vi "AlliGator Get Background Subtraction Parameters.vi"(6 "Get (F)/Set":bool, 8 "Error In":errorcluster, 11 "Background Subtraction Parameters in":T1={"Background Definition Range"={"Min Gate"=0.0, "Max Gate"=0.0}, "Baseline Subtraction Method"=enum."Mean", "Background Subtraction?"=FALSE, "Background File"=path "", "Background Constant"=0.0, "Background Scaling Factor"=1.0, "Background Pile-up Correction"=FALSE, "Background Pixel Well Capacity"=1} {"Background Pixel Well Capacity" min=1 step=1}) -> (0 "Error Out":errorcluster, 3 "Background Subtraction Parameters out":T1={"Background Definition Range"={"Min Gate"=0.0, "Max Gate"=0.0}, "Baseline Subtraction Method"=enum."Mean", "Background Subtraction?"=FALSE, "Background File"=path "", "Background Constant"=0.0, "Background Scaling Factor"=1.0, "Background Pile-up Correction"=FALSE, "Background Pixel Well Capacity"=1} {"Background Pixel Well Capacity" min=1 step=1})   [LabVIEW 2021, in "AlliGator Decay Preprocessing.lvlib"]
doc: "Obtains or stores information about <B>Background Subtraction Parameters</B> from Settings."
uses:
  AlliGator Decay Preprocessing.lvlib
  AlliGator Background Subtraction Parameters.ctl
  AlliGator Baseline Subtraction Method.ctl
  Settings/AlliGator Settings List.ctl
  Settings/AlliGator Settings.lvlib
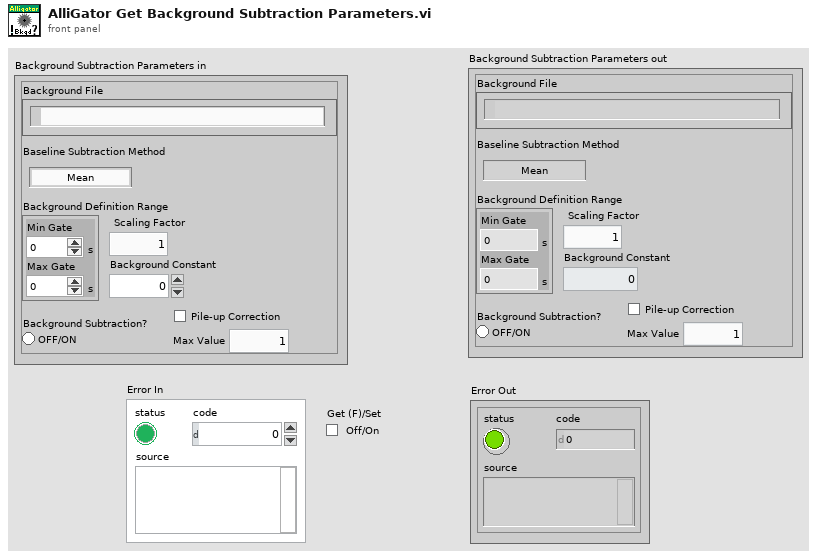
[diagram p1: front panel]
types:
  T1 = typedef "AlliGator Decay Preprocessing.lvlib/AlliGator Background Subtraction Parameters.ctl" = cluster{"Background Definition Range":cluster{"Min Gate":dbl[unit], "Max Gate":dbl[unit]}, "Baseline Subtraction Method":T2, "Background Subtraction?":bool, "Background File":path, "Background Constant":dbl, "Background Scaling Factor":dbl, "Background Pile-up Correction":bool, "Background Pixel Well Capacity":u32}
  T2 = typedef "AlliGator Decay Preprocessing.lvlib/AlliGator Baseline Subtraction Method.ctl" = enum16{"Mean", "Min", "Square Gated Single-Exponential", "File", "Constant"}
  T3 = typedef "AlliGator Settings.lvlib/AlliGator Settings List.ctl" = enum16{"GUI:Visible Settings Tab", "GUI:Last Run Version", "Source Image:Use Image Histogram for Contrast", "Source Image:Low Count Pixels Rejection Options", "Source Image:High Count Pixels Rejection Options", "Source Image:Use Image Brightness", "Source Image:Blend Overlay with Image Background", "Source Image:Use Fixed ROI Diameter", "Source Image:ROI Diameter", "Source Image:ROI Center Color", "Source Image:Peak Threshold", "Source Image:Intensity Threshold", "Source Image:Image Binning Options", "Source Image:Image Smoothing Options", "Source Image:Image Histogram Active", "Source Image:Invert Binary Mask", "Source Image:Hot Pixel Removal", "Source Image:Overlay Analyzed ROI Center", "Source Image:Auto-Adjust Contrast", "Source Image:Histogram Lower Percentile", "Source Image:Histogram Upper Percentile", "Source Image:Save Source Image", "Source Image:Scale Bar Options", "Source Image:Image Resolution (Pixel Size)", "Source Image:Flatfield Correction", "Source Image:Show Dead Left Columns Correction", "Source Image:Dead Left Columns Correction", "Source Image:Image Pre-Processing Operations Order", "Source Image:Overlay ROI Median", "Source Image:Median Overlay Color", "Data Information:Gate Width", "Data Information:Nanotime Gate Separation", "Data Information:Macrotime Gate Separation", "Data Information:Gate Step", "Data Information:# Gates", "Data Information:Gate Image Exposure", "Data Information:Gate Image Integration", "Data Information:Gates to Skip", "Data Information:Gates to Keep", "Data Information:Define Gates to", "Data Information:Channel Name", "Data Information:Available Channel Names", "Data Information:Channel Arithmetic", "Data Information:Background File Subtraction", "Data Information:Background File", "Data Information:Background Scaling Factor", "Data Information:Background Pile-up Correction", "Data Information:Background Pixel Well Capacity", "Data Information:Laser Period", "Data Information:SYNC Period", "Data Information:Pile-up Correction", "Data Information:Pixel Well Capacity", "Data Information:Dataset Scaling Factor", "Fluorescence Decay_Decay Pre-Processing:Reverse Gates", "Fluorescence Decay_Decay Pre-Processing:Verbose Decay Pre-Processing", "Fluorescence Decay_Decay Pre-Processing:Use Decay Pre-Processing", "Fluorescence Decay_Decay Pre-Processing:Background Subtraction", "Fluorescence Decay_Decay Pre-Processing:Background Definition Range", "Fluorescence Decay_Decay Pre-Processing:Baseline Subtraction Method", "Fluorescence Decay_Decay Pre-Processing:Decay Pre-Processing Operations Order", "Fluorescence Decay_Decay Pre-Processing:Smoothing Parameter", "Fluorescence Decay_Decay Pre-Processing:Shift Decay", "Fluorescence Decay_Decay Pre-Processing:Decay Shift Parameters", "Fluorescence Decay_Decay Pre-Processing:Fold Decay", "Fluorescence Decay_Decay Pre-Processing:# Folds", "Fluorescence Decay_Decay Pre-Processing:1-Normalize Decay", "Fluorescence Decay_Decay Pre-Processing:[0-1]-Normalize Decay", "Fluorescence Decay_Decay Pre-Processing:Smoothen Decay", "Fluorescence Decay_Decay Pre-Processing:Extrapolate Decay", "Fluorescence Decay_Decay Pre-Processing:Use Periodicity", "Fluorescence Decay_Decay Pre-Processing:Use Cursors", "Fluorescence Decay_Decay Pre-Processing:Tail Fraction", "Fluorescence Decay_Decay Pre-Processing:Head Fraction", "Fluorescence Decay_Decay Pre-Processing:Additional Points", "Fluorescence Decay_Decay Pre-Processing:Straighten Decay", "Fluorescence Decay_Decay Pre-Processing:Constant Background", "Fluorescence Decay_Decay Pre-Processing:Pixel-Normalize Decay", "Fluorescence Decay_Advanced Analysis:Extract IRF instead of Decay", "Fluorescence Decay_Advanced Analysis:IRF Extraction Options", "Fluorescence Decay_Advanced Analysis:IRF Optimization Options", "Fluorescence Decay_Advanced Analysis:Square Pulse Options", "Fluorescence Decay_Advanced Analysis:IRF Order", "Fluorescence Decay_Advanced Analysis:IRF Time Constants", "Fluorescence Decay_Advanced Analysis:Wavelet Analysis Options", "Fluorescence Decay_Advanced Analysis:Average Lifetime Options", "Fluorescence Decay_Fit Options:Fit Options", "Fluorescence Decay_Fit Options:Use Legacy Fitting Approach", "Fluorescence Decay_Fit Options:Use Data Information Laser Period", "Fluorescence Decay_Fit Parameters:Displayed Fit Parameters", "Fluorescence Decay_Fit Parameters:Fit Parameter Constraints", "Fluorescence Decay_Fit Parameters:Export Tabulated Results", "Fluorescence Decay_Fit Parameters:MLE Baseline Offset Type", "Fluorescence Decay_Fit Parameters:MLE Baseline Offset", "Fluorescence Decay_Fit Parameters:Guess Parameter Names", "Fluorescence Decay_Fit Parameters:Guess Parameter Values", "Fluorescence Decay_Fit Parameters:Guess Parameters Options", "Fluorescence Decay_Styles:Show Last Decay Only", "Fluorescence Decay_Styles:Decay Graph Color Array", "Fluorescence Decay:Decay Graph Active", "Fluorescence Decay Statistics:Min Peak Value", "Fluorescence Decay Statistics:Reject Low Decay Peak Pixels", "Fluorescence Decay Statistics:Reject High Decay Peak Pixels", "Fluorescence Decay Statistics:Max Peak Value", "Time Traces:Use File Timestamp", "Time Traces:Time Step", "Time Traces:Use Intensity Correction File", "Time Traces:Intensity Correction File", "Phasor Plot:Phasor Plot Smoothing Options", "Phasor Plot:Phasor Plot Size", "Phasor Plot:Phasor Plot Graphics Options", "Phasor Plot:Cumulative Phasor Plot", "Phasor Plot:Use Phasor Brightness", "Phasor Plot:Blend Overlay with Phasor Background", "Phasor Plot:Save Phasor Plot", "Phasor Plot:Show References", "Phasor Plot:Phasor Ratio Decay Range", "Phasor Plot:Exponential Fading", "Phasor Plot:Phasor Ratio Reference Colors", "Phasor Plot:Reference Radius", "Phasor Plot:Show Color Map Vertices", "Phasor Plot:Phasor Plot Active", "Phasor Plot:Phasor Ratio Color Map Type", "Phasor Plot:Phasor Ratio Color Map", "Phasor Plot:Phasor Ratio Display Range", "Phasor Plot:Selected Image ROI(s)", "Phasor Plot:All Image ROIs", "Phasor Plot:Selected Phasor Plot ROI(s)", "Phasor Plot:All Phasor Plot ROIs", "Phasor Plot:Phasor Ratio Color-Coded Quantity", "Phasor Plot:Store Phasor Harmonics", "Phasor Plot:Draw Reference Segment", "Phasor Plot:User-Defined Quantity", "Phasor Graph:Phasor Frequency", "Phasor Graph:Phasor Ratio Type", "Phasor Graph:Pixel-level Phasor Computation", "Phasor Graph:Save Phasor Graph", "Phasor Graph:Phasor Graph Active", "Phasor Graph:Phasor SDV Options", "Phasor Calibration:Use Backup Calibration if needed", "Phasor Graph:Define Shortest Lifetime as", "Phasor Calibration:Backup Calibration Type", "Phasor Calibration:Calibration Type", "Phasor Calibration:Calibration Lifetime", "Phasor Calibration:Calibration Map Algorithm", "Single-Exponential Phasor Locus (SEPL):Gate Parameters", "Single-Exponential Phasor Locus (SEPL):User-defined Gate", "Single-Exponential Phasor Locus (SEPL):User-defined IRF", "Single-Exponential Phasor Locus (SEPL):Phasor Parameters", "Single-Exponential Phasor Locus (SEPL):Decay & IRF Parameters", "Single-Exponential Phasor Locus (SEPL):Display Parameters", "Lifetime Analysis:Decay Analysis Parameters", "Lifetime Analysis:Lifetime Map Active", "Plugins:Python Settings", "Miscellaneous:Verbose Mode", "Miscellaneous:Beep after Script", "Miscellaneous:Saved Image File Format", "Miscellaneous:Exported Gate Image Settings", "Miscellaneous:Include Loading in Timing", "Miscellaneous:Verbose Settings Mode", "Miscellaneous:Histogram Options", "Miscellaneous:Beep on Error", "Miscellaneous:# Logical Processors Used", "Miscellaneous:ROI Description Max Characters", "Miscellaneous:Verbose Error Mode", "Miscellaneous:Transparent Mask Color"}
  T4 = cluster{"Min Gate":dbl[unit], "Max Gate":dbl[unit]}
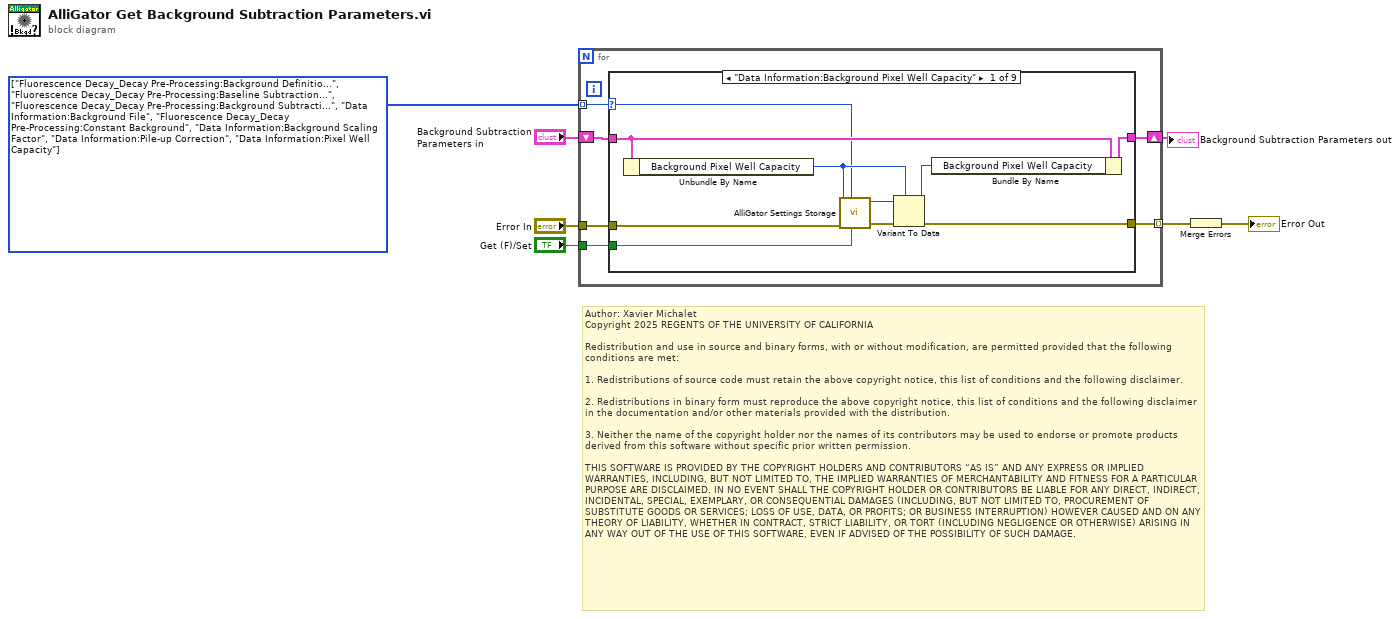
[diagram p0: block diagram]
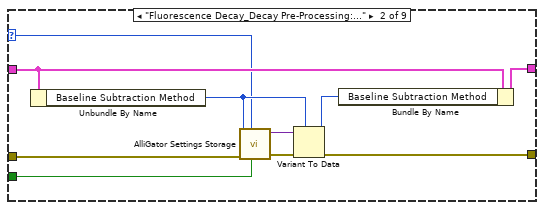
[diagram p2: hidden frame]
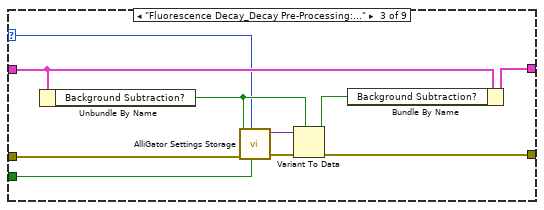
[diagram p3: hidden frame]
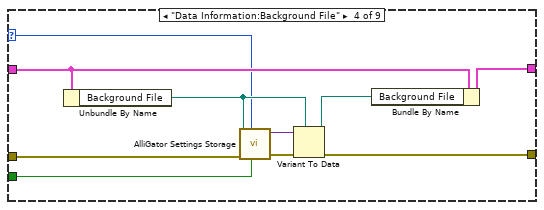
[diagram p4: hidden frame]
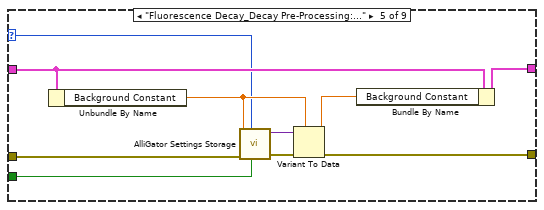
[diagram p5: hidden frame]
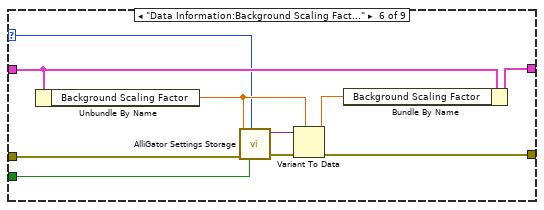
[diagram p6: hidden frame]
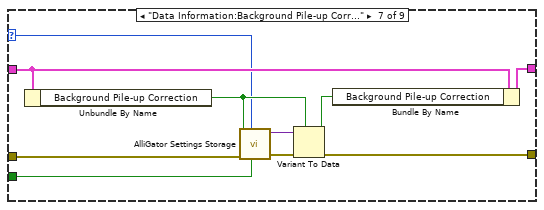
[diagram p7: hidden frame]
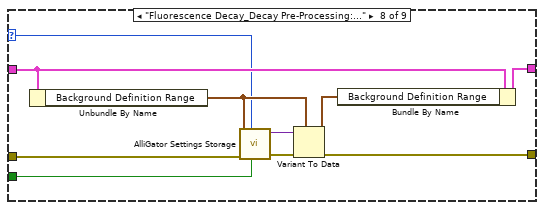
[diagram p8: hidden frame]
diagram:
  w1 = T3[] [enum."Fluorescence Decay_Decay Pre-Processing:Background Definition Range", enum."Fluorescence Decay_Decay Pre-Processing:Baseline Subtraction Method", enum."Fluorescence Decay_Decay Pre-Processing:Background Subtraction", enum."Data Information:Background File", enum."Fluorescence Decay_Decay Pre-Processing:Constant Background", enum."Data Information:Background Scaling Factor", enum."Data Information:Pile-up Correction", enum."Data Information:Pixel Well Capacity"] items=["GUI:Visible Settings Tab", "GUI:Last Run Version", "Source Image:Use Image Histogram for Contrast", "Source Image:Low Count Pixels Rejection Options", "Source Image:High Count Pixels Rejection Options", "Source Image:Use Image Brightness", "Source Image:Blend Overlay with Image Background", "Source Image:Use Fixed ROI Diameter", "Source Image:ROI Diameter", "Source Image:ROI Center Color", "Source Image:Peak Threshold", "Source Image:Intensity Threshold", "Source Image:Image Binning Options", "Source Image:Image Smoothing Options", "Source Image:Image Histogram Active", "Source Image:Invert Binary Mask", "Source Image:Hot Pixel Removal", "Source Image:Overlay Analyzed ROI Center", "Source Image:Auto-Adjust Contrast", "Source Image:Histogram Lower Percentile", "Source Image:Histogram Upper Percentile", "Source Image:Save Source Image", "Source Image:Scale Bar Options", "Source Image:Image Resolution (Pixel Size)", "Source Image:Flatfield Correction", "Source Image:Show Dead Left Columns Correction", "Source Image:Dead Left Columns Correction", "Source Image:Image Pre-Processing Operations Order", "Source Image:Overlay ROI Median", "Source Image:Median Overlay Color", "Data Information:Gate Width", "Data Information:Nanotime Gate Separation", "Data Information:Macrotime Gate Separation", "Data Information:Gate Step", "Data Information:# Gates", "Data Information:Gate Image Exposure", "Data Information:Gate Image Integration", "Data Information:Gates to Skip", "Data Information:Gates to Keep", "Data Information:Define Gates to", "Data Information:Channel Name", "Data Information:Available Channel Names", "Data Information:Channel Arithmetic", "Data Information:Background File Subtraction", "Data Information:Background File", "Data Information:Background Scaling Factor", "Data Information:Background Pile-up Correction", "Data Information:Background Pixel Well Capacity", "Data Information:Laser Period", "Data Information:SYNC Period", "Data Information:Pile-up Correction", "Data Information:Pixel Well Capacity", "Data Information:Dataset Scaling Factor", "Fluorescence Decay_Decay Pre-Processing:Reverse Gates", "Fluorescence Decay_Decay Pre-Processing:Verbose Decay Pre-Processing", "Fluorescence Decay_Decay Pre-Processing:Use Decay Pre-Processing", "Fluorescence Decay_Decay Pre-Processing:Background Subtraction", "Fluorescence Decay_Decay Pre-Processing:Background Definition Range", "Fluorescence Decay_Decay Pre-Processing:Baseline Subtraction Method", "Fluorescence Decay_Decay Pre-Processing:Decay Pre-Processing Operations Order", "Fluorescence Decay_Decay Pre-Processing:Smoothing Parameter", "Fluorescence Decay_Decay Pre-Processing:Shift Decay", "Fluorescence Decay_Decay Pre-Processing:Decay Shift Parameters", "Fluorescence Decay_Decay Pre-Processing:Fold Decay", "Fluorescence Decay_Decay Pre-Processing:# Folds", "Fluorescence Decay_Decay Pre-Processing:1-Normalize Decay", "Fluorescence Decay_Decay Pre-Processing:[0-1]-Normalize Decay", "Fluorescence Decay_Decay Pre-Processing:Smoothen Decay", "Fluorescence Decay_Decay Pre-Processing:Extrapolate Decay", "Fluorescence Decay_Decay Pre-Processing:Use Periodicity", "Fluorescence Decay_Decay Pre-Processing:Use Cursors", "Fluorescence Decay_Decay Pre-Processing:Tail Fraction", "Fluorescence Decay_Decay Pre-Processing:Head Fraction", "Fluorescence Decay_Decay Pre-Processing:Additional Points", "Fluorescence Decay_Decay Pre-Processing:Straighten Decay", "Fluorescence Decay_Decay Pre-Processing:Constant Background", "Fluorescence Decay_Decay Pre-Processing:Pixel-Normalize Decay", "Fluorescence Decay_Advanced Analysis:Extract IRF instead of Decay", "Fluorescence Decay_Advanced Analysis:IRF Extraction Options", "Fluorescence Decay_Advanced Analysis:IRF Optimization Options", "Fluorescence Decay_Advanced Analysis:Square Pulse Options", "Fluorescence Decay_Advanced Analysis:IRF Order", "Fluorescence Decay_Advanced Analysis:IRF Time Constants", "Fluorescence Decay_Advanced Analysis:Wavelet Analysis Options", "Fluorescence Decay_Advanced Analysis:Average Lifetime Options", "Fluorescence Decay_Fit Options:Fit Options", "Fluorescence Decay_Fit Options:Use Legacy Fitting Approach", "Fluorescence Decay_Fit Options:Use Data Information Laser Period", "Fluorescence Decay_Fit Parameters:Displayed Fit Parameters", "Fluorescence Decay_Fit Parameters:Fit Parameter Constraints", "Fluorescence Decay_Fit Parameters:Export Tabulated Results", "Fluorescence Decay_Fit Parameters:MLE Baseline Offset Type", "Fluorescence Decay_Fit Parameters:MLE Baseline Offset", "Fluorescence Decay_Fit Parameters:Guess Parameter Names", "Fluorescence Decay_Fit Parameters:Guess Parameter Values", "Fluorescence Decay_Fit Parameters:Guess Parameters Options", "Fluorescence Decay_Styles:Show Last Decay Only", "Fluorescence Decay_Styles:Decay Graph Color Array", "Fluorescence Decay:Decay Graph Active", "Fluorescence Decay Statistics:Min Peak Value", "Fluorescence Decay Statistics:Reject Low Decay Peak Pixels", "Fluorescence Decay Statistics:Reject High Decay Peak Pixels", "Fluorescence Decay Statistics:Max Peak Value", "Time Traces:Use File Timestamp", "Time Traces:Time Step", "Time Traces:Use Intensity Correction File", "Time Traces:Intensity Correction File", "Phasor Plot:Phasor Plot Smoothing Options", "Phasor Plot:Phasor Plot Size", "Phasor Plot:Phasor Plot Graphics Options", "Phasor Plot:Cumulative Phasor Plot", "Phasor Plot:Use Phasor Brightness", "Phasor Plot:Blend Overlay with Phasor Background", "Phasor Plot:Save Phasor Plot", "Phasor Plot:Show References", "Phasor Plot:Phasor Ratio Decay Range", "Phasor Plot:Exponential Fading", "Phasor Plot:Phasor Ratio Reference Colors", "Phasor Plot:Reference Radius", "Phasor Plot:Show Color Map Vertices", "Phasor Plot:Phasor Plot Active", "Phasor Plot:Phasor Ratio Color Map Type", "Phasor Plot:Phasor Ratio Color Map", "Phasor Plot:Phasor Ratio Display Range", "Phasor Plot:Selected Image ROI(s)", "Phasor Plot:All Image ROIs", "Phasor Plot:Selected Phasor Plot ROI(s)", "Phasor Plot:All Phasor Plot ROIs", "Phasor Plot:Phasor Ratio Color-Coded Quantity", "Phasor Plot:Store Phasor Harmonics", "Phasor Plot:Draw Reference Segment", "Phasor Plot:User-Defined Quantity", "Phasor Graph:Phasor Frequency", "Phasor Graph:Phasor Ratio Type", "Phasor Graph:Pixel-level Phasor Computation", "Phasor Graph:Save Phasor Graph", "Phasor Graph:Phasor Graph Active", "Phasor Graph:Phasor SDV Options", "Phasor Calibration:Use Backup Calibration if needed", "Phasor Graph:Define Shortest Lifetime as", "Phasor Calibration:Backup Calibration Type", "Phasor Calibration:Calibration Type", "Phasor Calibration:Calibration Lifetime", "Phasor Calibration:Calibration Map Algorithm", "Single-Exponential Phasor Locus (SEPL):Gate Parameters", "Single-Exponential Phasor Locus (SEPL):User-defined Gate", "Single-Exponential Phasor Locus (SEPL):User-defined IRF", "Single-Exponential Phasor Locus (SEPL):Phasor Parameters", "Single-Exponential Phasor Locus (SEPL):Decay & IRF Parameters", "Single-Exponential Phasor Locus (SEPL):Display Parameters", "Lifetime Analysis:Decay Analysis Parameters", "Lifetime Analysis:Lifetime Map Active", "Plugins:Python Settings", "Miscellaneous:Verbose Mode", "Miscellaneous:Beep after Script", "Miscellaneous:Saved Image File Format", "Miscellaneous:Exported Gate Image Settings", "Miscellaneous:Include Loading in Timing", "Miscellaneous:Verbose Settings Mode", "Miscellaneous:Histogram Options", "Miscellaneous:Beep on Error", "Miscellaneous:# Logical Processors Used", "Miscellaneous:ROI Description Max Characters", "Miscellaneous:Verbose Error Mode", "Miscellaneous:Transparent Mask Color"] ("Array")
  # "Author: Xavier Michalet\nCopyright 2025 REGENTS OF THE UNIVERSITY OF CALIFORNIA\n\nRedistribution and use in source and binary forms, with or without modification, are permitted provided that the following conditions are met:\n\n1. Redistributions of source code must retain the above copyright notice, this list of conditions and the following disclaimer.\n\n2. Redistributions in binary form must reproduce the above copyright notice, this list of conditions and the following disclaimer in the documentation and/or other materials provided with the distribution.\n\n3. Neither the name of the copyright holder nor the names of its contributors may be used to endorse or promote products derived from this software without specific prior written permission.\n\nTHIS SOFTWARE IS PROVIDED BY THE COPYRIGHT HOLDERS AND CONTRIBUTORS “AS IS” AND ANY EXPRESS OR IMPLIED WARRANTIES, INCLUDING, BUT NOT LIMITED TO, THE IMPLIED WARRANTIES OF MERCHANTABILITY AND FITNESS FOR A PARTICULAR PURPOSE ARE DISCLAIMED. IN NO EVENT SHALL THE COPYRIGHT HOLDER OR CONTRIBUTORS BE LIABLE FOR ANY DIRECT, INDIRECT, INCIDENTAL, SPECIAL, EXEMPLARY, OR CONSEQUENTIAL DAMAGES (INCLUDING, BUT NOT LIMITED TO, PROCUREMENT OF SUBSTITUTE GOODS OR SERVICES; LOSS OF USE, DATA, OR PROFITS; OR BUSINESS INTERRUPTION) HOWEVER CAUSED AND ON ANY THEORY OF LIABILITY, WHETHER IN CONTRACT, STRICT LIABILITY, OR TORT (INCLUDING NEGLIGENCE OR OTHERWISE) ARISING IN ANY WAY OUT OF THE USE OF THIS SOFTWARE, EVEN IF ADVISED OF THE POSSIBILITY OF SUCH DAMAGE."
  n1 = for {
    shift-right: [w12] -> w6
    shift-left: "Background Subtraction Parameters in" -> [w13]
    tunnel: "Error In" -> [w11]
    tunnel: [w10] -> w5 mode=indexing
    tunnel: "Get (F)/Set" -> [w9]
    tunnel: w1 -> [w8] mode=indexing
    n2 = case shown="\"Data Information:Background Pixel Well Capacity\"" w8 {
      selector: w8 -> [w14 w24 w34 w44 w54 w64 w74 w84 _]
      tunnel: w13 -> [w21 w31 w41 w51 w61 w71 w81 w91 w95]
      tunnel: [w18 w28 w38 w48 w58 w68 w78 w88 w95] -> w12
      tunnel: w11 -> [w17 w27 w37 w47 w57 w67 w77 w87 w94]
      tunnel: [w16 w26 w35 w46 w56 w66 w76 w86 w94] -> w10
      tunnel: w9 -> [w15 w25 w36 w45 w55 w65 w75 w85 _]
      frame "Data Information:Background Pixel Well Capacity" {
        n3 = Unbundle By Name(w21) -> ("Background Pixel Well Capacity"=w19:u32)
        n4 = call "AlliGator Settings Storage.vi"("Get(F)/Set"=w15, "AlliGator Settings List"=w14, "Error In"=w17, "Variant Data in"=w19) -> ("Error Out"=w23:errorcluster, "Variant Data out"=w22:variant)  [unwired: 6 in]
        n5 = Variant To Data(error in=w23, type=w19, Variant=w22) -> (data=w20:u32, error out=w16:errorcluster)
        n6 = Bundle By Name(cluster=w21, "Background Pixel Well Capacity"=w20) -> (w18:T1)
      }
      frame "Fluorescence Decay_Decay Pre-Processing:Baseline Subtraction Method" {
        n7 = Unbundle By Name(w31) -> ("Baseline Subtraction Method"=w29:T2)
        n8 = call "AlliGator Settings Storage.vi"("Get(F)/Set"=w25, "AlliGator Settings List"=w24, "Error In"=w27, "Variant Data in"=w29) -> ("Error Out"=w33:errorcluster, "Variant Data out"=w32:variant)  [unwired: 6 in]
        n9 = Variant To Data(error in=w33, type=w29, Variant=w32) -> (data=w30:T2, error out=w26:errorcluster)
        n10 = Bundle By Name(cluster=w31, "Baseline Subtraction Method"=w30) -> (w28:T1)
      }
      frame "Fluorescence Decay_Decay Pre-Processing:Background Subtraction" {
        n11 = Unbundle By Name(w41) -> ("Background Subtraction?"=w39:bool)
        n12 = call "AlliGator Settings Storage.vi"("Get(F)/Set"=w36, "AlliGator Settings List"=w34, "Error In"=w37, "Variant Data in"=w39) -> ("Error Out"=w43:errorcluster, "Variant Data out"=w42:variant)  [unwired: 6 in]
        n13 = Variant To Data(error in=w43, type=w39, Variant=w42) -> (data=w40:bool, error out=w35:errorcluster)
        n14 = Bundle By Name(cluster=w41, "Background Subtraction?"=w40) -> (w38:T1)
      }
      frame "Data Information:Background File" {
        n15 = Unbundle By Name(w51) -> ("Background File"=w49:path)
        n16 = call "AlliGator Settings Storage.vi"("Get(F)/Set"=w45, "AlliGator Settings List"=w44, "Error In"=w47, "Variant Data in"=w49) -> ("Error Out"=w53:errorcluster, "Variant Data out"=w52:variant)  [unwired: 6 in]
        n17 = Variant To Data(error in=w53, type=w49, Variant=w52) -> (data=w50:path, error out=w46:errorcluster)
        n18 = Bundle By Name(cluster=w51, "Background File"=w50) -> (w48:T1)
      }
      frame "Fluorescence Decay_Decay Pre-Processing:Constant Background" {
        n19 = Unbundle By Name(w61) -> ("Background Constant"=w59:dbl)
        n20 = call "AlliGator Settings Storage.vi"("Get(F)/Set"=w55, "AlliGator Settings List"=w54, "Error In"=w57, "Variant Data in"=w59) -> ("Error Out"=w63:errorcluster, "Variant Data out"=w62:variant)  [unwired: 6 in]
        n21 = Variant To Data(error in=w63, type=w59, Variant=w62) -> (data=w60:dbl, error out=w56:errorcluster)
        n22 = Bundle By Name(cluster=w61, "Background Constant"=w60) -> (w58:T1)
      }
      frame "Data Information:Background Scaling Factor" {
        n23 = Unbundle By Name(w71) -> ("Background Scaling Factor"=w69:dbl)
        n24 = call "AlliGator Settings Storage.vi"("Get(F)/Set"=w65, "AlliGator Settings List"=w64, "Error In"=w67, "Variant Data in"=w69) -> ("Error Out"=w73:errorcluster, "Variant Data out"=w72:variant)  [unwired: 6 in]
        n25 = Variant To Data(error in=w73, type=w69, Variant=w72) -> (data=w70:dbl, error out=w66:errorcluster)
        n26 = Bundle By Name(cluster=w71, "Background Scaling Factor"=w70) -> (w68:T1)
      }
      frame "Data Information:Background Pile-up Correction" {
        n27 = Unbundle By Name(w81) -> ("Background Pile-up Correction"=w79:bool)
        n28 = call "AlliGator Settings Storage.vi"("Get(F)/Set"=w75, "AlliGator Settings List"=w74, "Error In"=w77, "Variant Data in"=w79) -> ("Error Out"=w83:errorcluster, "Variant Data out"=w82:variant)  [unwired: 6 in]
        n29 = Variant To Data(error in=w83, type=w79, Variant=w82) -> (data=w80:bool, error out=w76:errorcluster)
        n30 = Bundle By Name(cluster=w81, "Background Pile-up Correction"=w80) -> (w78:T1)
      }
      frame "Fluorescence Decay_Decay Pre-Processing:Background Definition Range" {
        n31 = Unbundle By Name(w91) -> ("Background Definition Range"=w89:T4)
        n32 = call "AlliGator Settings Storage.vi"("Get(F)/Set"=w85, "AlliGator Settings List"=w84, "Error In"=w87, "Variant Data in"=w89) -> ("Error Out"=w93:errorcluster, "Variant Data out"=w92:variant)  [unwired: 6 in]
        n33 = Variant To Data(error in=w93, type=w89, Variant=w92) -> (data=w90:T4, error out=w86:errorcluster)
        n34 = Bundle By Name(cluster=w91, "Background Definition Range"=w90) -> (w88:T1)
      }
      frame "Fluorescence Decay_Decay Pre-Processing:Decay Pre-Processing Operations Order", Default {
      }
    }
  }
  "Background Subtraction Parameters out" <- w6
  n35 = Merge Errors(w5) -> (→"Error Out":errorcluster)
